vi "Untitled 2.vi"() -> ()   [LabVIEW 2014]
panel:
  in  "Array":bool[](array[boolean])
  in  "Enum":enum16{"", "1", "2", "3", "4", "5", "6", "7"}(ring)
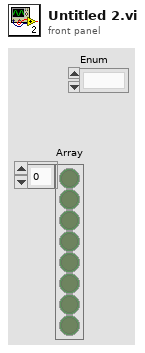
[diagram p1: front panel]
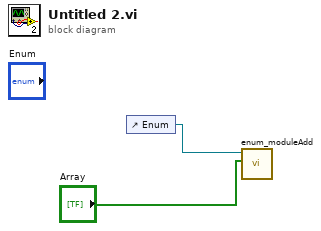
[diagram p0: block diagram]
diagram:
  n1 = control-ref of="Enum"() -> (w2:refnum<vi>)
  n2 = call "enum_moduleAdd.vi"("in_modules"="Array", "enum_refin"=w2) -> ()  [unwired: 9 in, 1 out]
